vi "set_reference_object.vi"(1 "camera cluster":T2, 2 "bit depth":i32) -> (0 "last acquired buffer out":i32)   [LabVIEW 2010]
uses:
  <vilib>/userDefined/High Color/IMAQdx.ctl
  MWT_1.3.0_r1035/MultiWorm Tracker v1.3.0/data/MWT.dll
panel:
  in  "Store Reference Object from image":bool
  out "initial frame number":i32
  out "Reference Object Image":T3(plugin-control)
  in  "Reset":bool
  in  "Set":bool
  in  "Cancel":bool
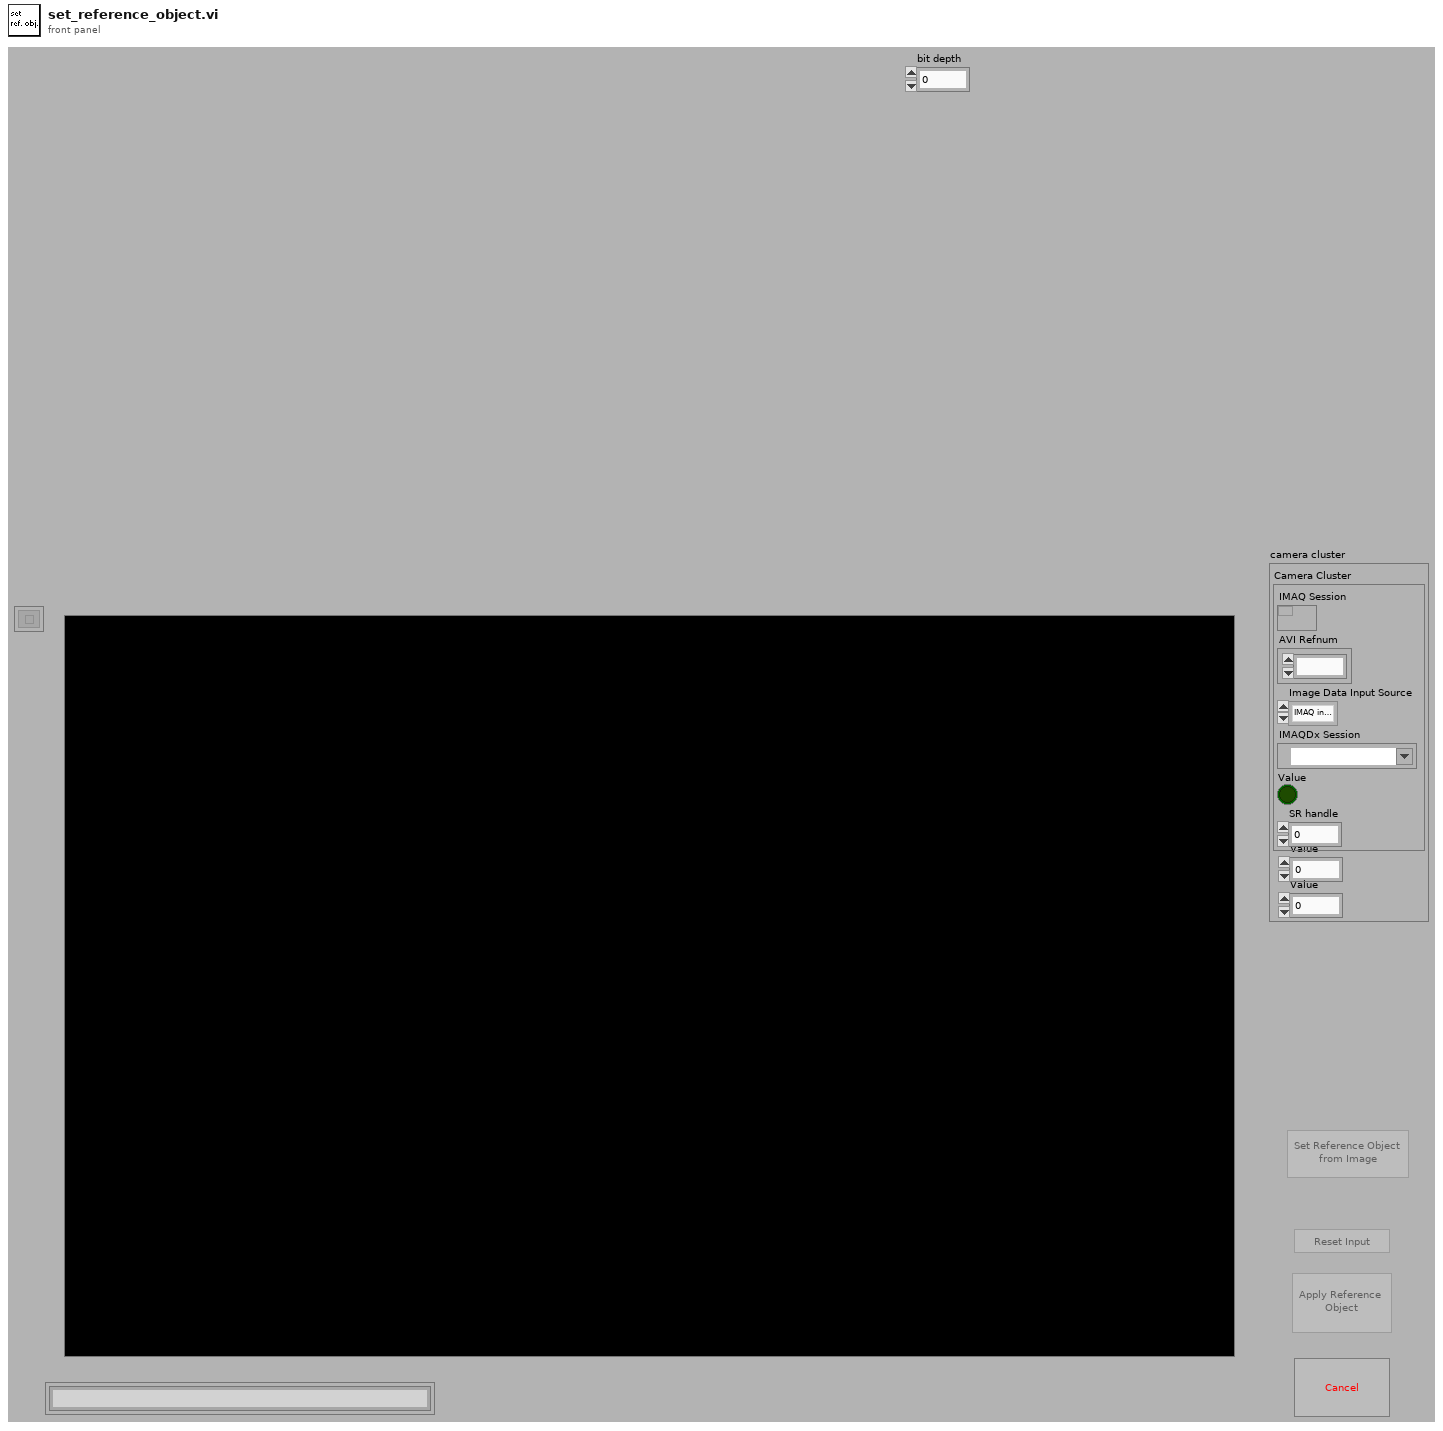
[diagram p1: front panel]
types:
  T1 = typedef "IMAQdx.ctl" = refnum<k21>
  T2 = cluster{"Camera Cluster":cluster{"IMAQ Session":refnum<k11>, "AVI Refnum":refnum<k1>, "Image Data Input Source":enum32{"IMAQ interface", "IMAQdx interface", "AVI file", "MMF File"}, "IMAQDx Session":T1, "Value":bool, "SR handle":u32}, "Value":i32, "Value":i32}
  T3 = typedef "IMAQ Image.ctl" = refnum<image>
  T4 = cluster{"Global Rectangle":i32[], "Contours":cluster{"Contour Type":u32, "ROI Type":u32, "Points":i32[]}[]}
  T5 = enum8{"Enabled", "Disabled", "Disabled and Grayed Out"}
  T6 = cluster{"IMAQ Session":refnum<k11>, "AVI Refnum":refnum<k1>, "Image Data Input Source":enum32{"IMAQ interface", "IMAQdx interface", "AVI file", "MMF File"}, "IMAQDx Session":T1, "Value":bool, "SR handle":u32}
  T7 = cluster{"Camera Cluster":cluster{"IMAQ Session":refnum<k11>, "AVI Refnum":refnum<k1>, "Image Data Input Source":enum32{"IMAQ interface", "IMAQdx interface", "AVI file", "MMF File"}, "IMAQDx Session":T1, "Value":bool, "SR handle":u32}, "Value":i32}
  T8 = cluster{"Camera Cluster":cluster{"IMAQ Session":refnum<k11>, "AVI Refnum":refnum<k1>, "Image Data Input Source":enum32{"IMAQ interface", "IMAQdx interface", "AVI file", "MMF File"}, "IMAQDx Session":T1, "Value":bool, "SR handle":u32}, "Acquired Buffer Number":i32}
  T9 = cluster{"Value":i32, i32, i32, "Image Pixels (I16)":i16[][]}
  T10 = cluster{"Value":i32, "Image Pixels (I16)":i16[][], "Image Pixels (I16)":i16[][], "Image Area Height":u32, "Image Area Width":u32}
  T11 = cluster{"return type":i32, "return type":i32, "destination":i16[][]}
  T12 = enum32{"IMAQ interface", "IMAQdx interface", "AVI file", "MMF File"}
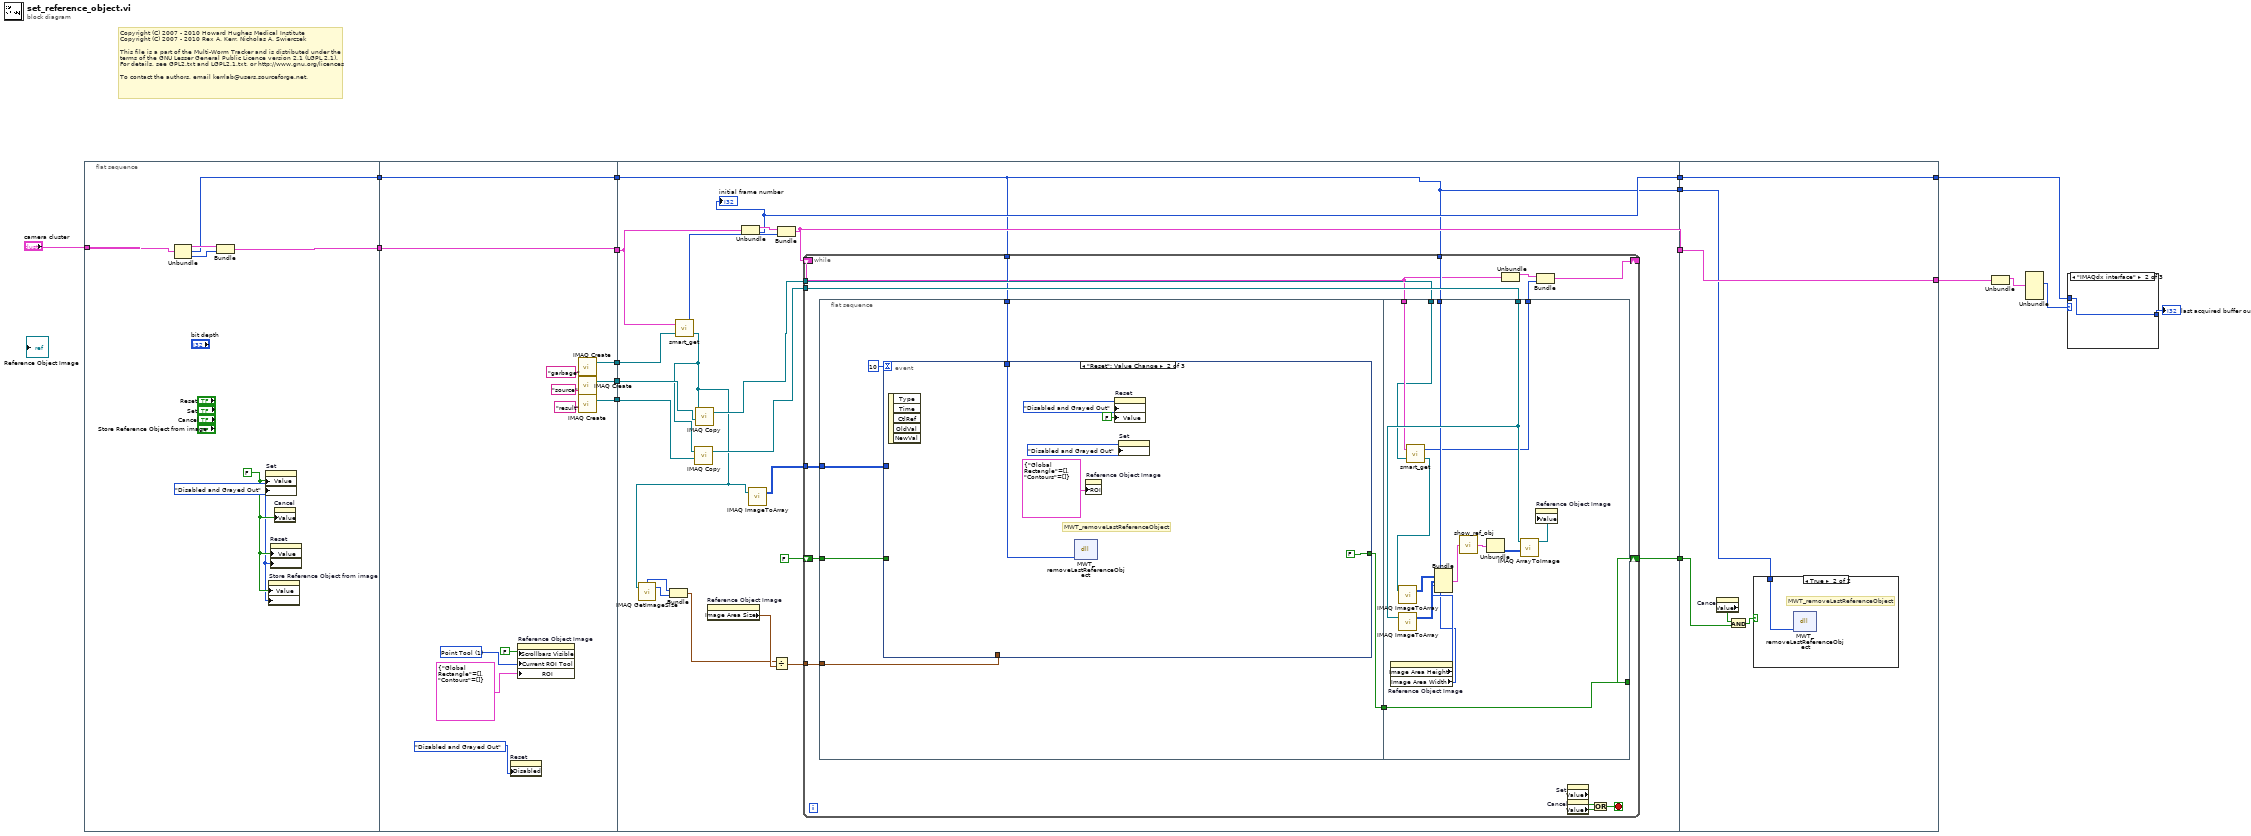
[diagram p0: block diagram]
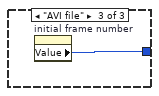
[diagram p3: hidden frame]
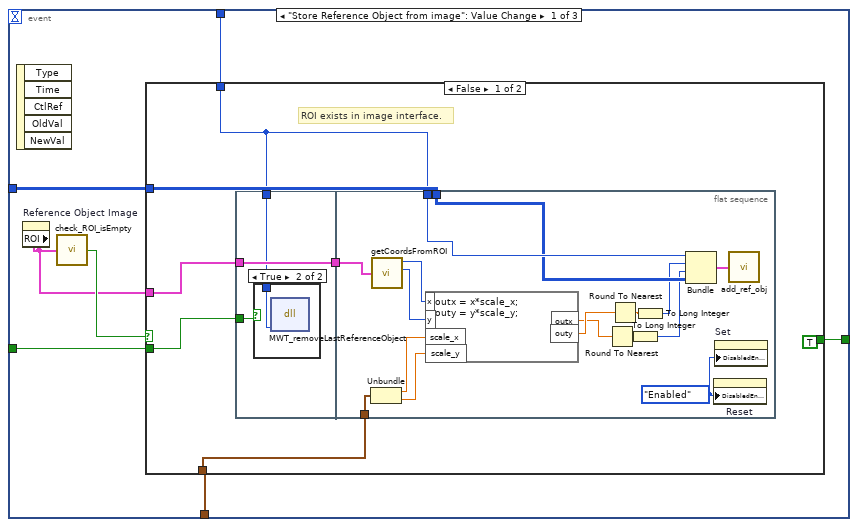
[diagram p4: hidden frame]
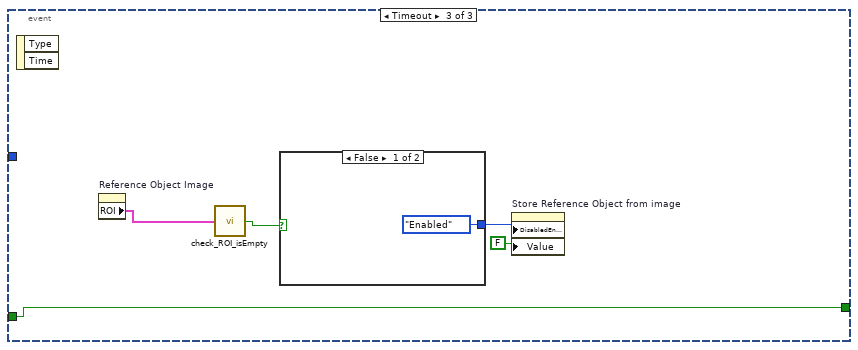
[diagram p7: hidden frame]
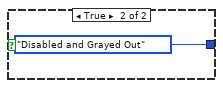
[diagram p8: hidden frame]
diagram:
  # "Copyright (C) 2007 - 2010 Howard Hughes Medical Institute\nCopyright (C) 2007 - 2010 Rex A. Kerr, Nicholas A. Swierczek\n \nThis file is a part of the Multi-Worm Tracker and is distributed under the\nterms of the GNU Lesser General Public Licence version 2.1 (LGPL 2.1).\nFor details, see GPL2.txt and LGPL2.1.txt, or http://www.gnu.org/licences\n \nTo contact the authors, email kerrlab@users.sourceforge.net."
  n1 = flat-sequence {
    tunnel: "camera cluster" -> [w24]
    tunnel: [w21] -> w17
    tunnel: [w20] -> w16
    tunnel: w17 -> [w31]
    tunnel: [w31] -> w14
    tunnel: [w35] -> w13
    tunnel: w16 -> [w35]
    tunnel: [w27] -> w6
    tunnel: [w26] -> w5
    tunnel: [w25] -> w4
    tunnel: w14 -> [w54]
    tunnel: w13 -> [w37]
    tunnel: [w53] -> w12
    tunnel: [w41] -> w11
    tunnel: w6 -> [w52]
    tunnel: w5 -> [w51]
    tunnel: w4 -> [w49]
    tunnel: [w38] -> w3
    tunnel: [w37] -> w2
    tunnel: w12 -> [w146]
    tunnel: w11 -> [w147]
    tunnel: [w147] -> w10
    tunnel: [w146] -> w7
    tunnel: w3 -> [w144]
    tunnel: w2 -> [w142]
    frame #0 {
      w18 = T5."Disabled and Grayed Out" ("Disabled")
      w19 = FALSE ("Set")
      n2 = Unbundle(w24) -> ("Camera Cluster"=w22:T6, "Value"=w20:i32, "Value"=w23:i32)
      n3 = Bundle("Camera Cluster"=w22, "Value"=w23) -> (w21:T7)  [unwired: 1 in]
      n4 = property on="Set" class="Bool (strict)"("Value"=w19, "DisabledEnum"=w18) -> ()  [unwired: 2 in, 2 out]
      n5 = property on="Store Reference Object from image" class="Bool (strict)"("Value"=w19, "DisabledEnum"=w18) -> ()  [unwired: 2 in, 2 out]
      n6 = property on="Reset" class="Bool (strict)"("Value"=w19, "DisabledEnum"=w18) -> ()  [unwired: 2 in, 2 out]
      n7 = property on="Cancel" class="Bool (strict)"("Value"=w19) -> ()  [unwired: 2 in, 2 out]
    }
    frame #1 {
      w34 = u32 1 items=["Zoom Tool"=8, "Selection Tool"=0, "Pan Tool"=9, "Point Tool"=1, "Line Tool"=2, "Rectangle Tool"=3, "Rotated Rectangle Tool"=12, "Polyline Tool"=10, "Polygon Tool"=5, "Freehand Tool"=11, "Closed Freehand Tool"=6, "Ellipse Tool"=4, "Annulus Tool"=7] ("Current ROI Tool")
      n8 = property on="Reset" class="Bool (strict)"("Disabled"=T5."Disabled and Grayed Out") -> ()  [unwired: 2 in, 2 out]
      n9 = property on="Reference Object Image" class="ImageControl"("Scrollbars Visible"=FALSE, "Current ROI Tool"=w34, "ROI"=T4 {"Global Rectangle"=[], "Contours"=[]}) -> ()  [unwired: 2 in, 2 out]
      n10 = call "IMAQ Create"("Image Name"="garbage") -> ("New Image"=w27:T3)  [unwired: 4 in, 1 out]
      n11 = call "IMAQ Create"("Image Name"="source") -> ("New Image"=w25:T3)  [unwired: 4 in, 1 out]
      n12 = call "IMAQ Create"("Image Name"="result") -> ("New Image"=w26:T3)  [unwired: 4 in, 1 out]
    }
    frame #2 {
      n13 = call "smart_get.vi"("Input Image"=w52, "Cluster"=w54) -> ("Image Out"=w43:T3, "Acquired Buffer Number"=w56:i32)
      n14 = call "IMAQ GetImageSize"("Image"=w43) -> ("Y Resolution"=w44:i32, "X Resolution"=w45:i32)  [unwired: 3 in, 1 out]
      n15 = Bundle("X Resolution"=w45, "Y Resolution"=w44) -> (w39:cluster{"X Resolution":i32, "Y Resolution":i32})  [unwired: 1 in]
      n16 = call "IMAQ Copy"("Image Dst"=w51, "Image Src"=w43) -> ("Image Dst Out"=w50:T3)  [unwired: 4 in, 1 out]
      n17 = call "IMAQ Copy"("Image Dst"=w49, "Image Src"=w43) -> ("Image Dst Out"=w48:T3)  [unwired: 4 in, 1 out]
      n18 = property on="Reference Object Image" class="ImageControl"() -> ("Image Area Size"=w40:cluster{"Width":u32, "Height":u32})  [unwired: 2 in, 2 out]
      n19 = Unbundle(w54) -> ("Camera Cluster"=w55:T6, "Value"=w53:i32)
      "initial frame number" <- w53
      n20 = call "IMAQ ImageToArray"("Image"=w43) -> ("Image Pixels (I16)"=w46:i16[][])  [unwired: 3 in, 4 out]
      n21 = Divide(x=w39, y=w40) -> (x/y=w42:cluster{dbl, dbl})
      n22 = Bundle("Camera Cluster"=w55, "Acquired Buffer Number"=w56) -> (w41:T8)  [unwired: 1 in]
      n23 = while {
        tunnel: w50 -> [w69]
        tunnel: w48 -> [w68]
        tunnel: w37 -> [w67]
        shift-right: [w64] -> w38
        shift-left: FALSE -> [w66]
        tunnel: w37 -> [w63]
        tunnel: w46 -> [w62]
        tunnel: w42 -> [w61]
        shift-right: [w57] -> _
        shift-left: w41 -> [w59]
        stop <- w70 stop-if-true
        n24 = flat-sequence {
          tunnel: w66 -> [w77]
          tunnel: [w76] -> w65
          tunnel: w63 -> [w75]
          tunnel: w62 -> [w74]
          tunnel: w61 -> [w73]
          tunnel: w69 -> [w138]
          tunnel: w68 -> [w128]
          tunnel: w67 -> [w137]
          tunnel: w65 -> [w131]
          tunnel: [w131] -> w64
          tunnel: w59 -> [w130]
          tunnel: [w129] -> w58
          frame #0 {
            n25 = event shown="[1] \"Reset\": Value Change" {
              selector: _ -> [_ _ _]
              dyn-events: _ -> [_ _ _]
              timeout: 10 -> [_ _ _]
              tunnel: w77 -> [w84 _ w124]
              tunnel: [w83 FALSE w124] -> w76
              tunnel: w75 -> [w81 w118 _]
              tunnel: w74 -> [w80 _ _]
              tunnel: w73 -> [w79 _ _]
              event "Store Reference Object from image": Value Change {
                n26 = event-data() -> ()  [unwired: 1 in, 5 out]
                n27 = property on="Reference Object Image" class="ImageControl"() -> ("ROI"=w82:T4)  [unwired: 2 in, 2 out]
                n28 = call "check_ROI_isEmpty.vi"("ROI"=w82) -> ("empty?"=w85:bool)
                n29 = case shown="False" w85 {
                  tunnel: w84 -> [w86 w113]
                  tunnel: [TRUE w113] -> w83
                  tunnel: w82 -> [w91 _]
                  tunnel: w81 -> [w87 _]
                  tunnel: w80 -> [w90 _]
                  tunnel: w79 -> [w89 _]
                  frame False {
                    # "ROI exists in image interface."
                    n30 = flat-sequence {
                      tunnel: w91 -> [w95]
                      tunnel: [w95] -> w88
                      tunnel: w87 -> [w94]
                      tunnel: w86 -> [w93]
                      tunnel: w87 -> [w111]
                      tunnel: w90 -> [w110]
                      tunnel: w89 -> [w109]
                      tunnel: w88 -> [w112]
                      frame #0 {
                        n31 = case shown="True" w93 {
                          tunnel: w94 -> [_ w96]
                          frame False {
                          }
                          frame True {
                            n32 = dll-call lib="C:/Users/Marc/multi worm tracker/MWT_1.3.0_r1035/MultiWorm Tracker v1.3.0/data/MWT.dll" fn="MWT_removeLastReferenceObject"("handle"=w96) -> ()  [unwired: 5 in, 2 out]
                          }
                        }
                      }
                      frame #1 {
                        w97 = T5."Enabled" ("Disabled")
                        n33 = Unbundle(w109) -> (w101:dbl, w100:dbl)
                        n34 = call "getCoordsFromROI.vi"("ROI"=w112) -> ("y1"=w102:i32, "x1"=w103:i32)  [unwired: 2 out]
                        n35 = formula code="outx = x*scale_x;\nouty = y*scale_y;"("x"=w103, "y"=w102, "scale_x"=w101, "scale_y"=w100) -> ("outx"=w98:dbl, "outy"=w99:dbl)
                        n36 = Round To Nearest(number=w98) -> (nearest integer value=w104:dbl)
                        n37 = Round To Nearest(number=w99) -> (nearest integer value=w105:dbl)
                        n38 = To Long Integer(number=w104) -> (32bit integer=w107:i32)
                        n39 = To Long Integer(number=w105) -> (32bit integer=w106:i32)
                        n40 = Bundle("Value"=w111, w106, w107, "Image Pixels (I16)"=w110) -> (w108:T9)  [unwired: 1 in]
                        n41 = property on="Reset" class="Bool (strict)"("DisabledEnum"=w97) -> ()  [unwired: 2 in, 2 out]
                        n42 = property on="Set" class="Bool (strict)"("DisabledEnum"=w97) -> ()  [unwired: 2 in, 2 out]
                        n43 = call "add_ref_obj.vi"("input cluster"=w108) -> ()  [unwired: 1 out]
                      }
                    }
                  }
                  frame True {
                    # "No ROI set in image interface.\nDo nothing."
                  }
                }
              }
              event "Reset": Value Change {
                # "MWT_removeLastReferenceObject"
                n44 = event-data() -> ()  [unwired: 1 in, 5 out]
                n45 = dll-call lib="C:/Users/Marc/multi worm tracker/MWT_1.3.0_r1035/MultiWorm Tracker v1.3.0/data/MWT.dll" fn="MWT_removeLastReferenceObject"("handle"=w118) -> ()  [unwired: 5 in, 2 out]
                n46 = property on="Reference Object Image" class="ImageControl"("ROI"=T4 {"Global Rectangle"=[], "Contours"=[]}) -> ()  [unwired: 2 in, 2 out]
                n47 = property on="Reset" class="Bool (strict)"("DisabledEnum"=T5."Disabled and Grayed Out" ("Disabled"), "Value"=FALSE ("Reset")) -> ()  [unwired: 2 in, 2 out]
                n48 = property on="Set" class="Bool (strict)"("DisabledEnum"=T5."Disabled and Grayed Out" ("Disabled")) -> ()  [unwired: 2 in, 2 out]
              }
              event Timeout {
                n49 = event-data() -> ()  [unwired: 1 in, 2 out]
                n50 = property on="Reference Object Image" class="ImageControl"() -> ("ROI"=w123:T4)  [unwired: 2 in, 2 out]
                n51 = call "check_ROI_isEmpty.vi"("ROI"=w123) -> ("empty?"=w122:bool)
                n52 = case shown="False" w122 {
                  tunnel: [T5."Enabled" ("Disabled") T5."Disabled and Grayed Out" ("Disabled")] -> w121
                  frame False {
                  }
                  frame True {
                  }
                }
                n53 = property on="Store Reference Object from image" class="Bool (strict)"("DisabledEnum"=w121, "Value"=FALSE ("Store Reference Object from image")) -> ()  [unwired: 2 in, 2 out]
              }
            }
          }
          frame #1 {
            n54 = property on="Reference Object Image" class="ImageControl"() -> ("Image Area Height"=w134:u32, "Image Area Width"=w133:u32)  [unwired: 2 in, 2 out]
            n55 = call "IMAQ ImageToArray"("Image"=w138) -> ("Image Pixels (I16)"=w135:i16[][])  [unwired: 3 in, 4 out]
            n56 = call "smart_get.vi"("Input Image"=w128, "Cluster"=w130) -> ("Image Out"=w127:T3, "Acquired Buffer Number"=w129:i32)
            n57 = call "IMAQ ImageToArray"("Image"=w127) -> ("Image Pixels (I16)"=w136:i16[][])  [unwired: 3 in, 4 out]
            n58 = Bundle("Value"=w137, "Image Pixels (I16)"=w136, "Image Pixels (I16)"=w135, "Image Area Height"=w134, "Image Area Width"=w133) -> (w132:T10)  [unwired: 1 in]
            n59 = call "show_ref_obj.vi"("input cluster"=w132) -> ("output cluster"=w141:T11)
            n60 = Unbundle(w141) -> ("destination"=w140:i16[][])  [unwired: 2 out]
            n61 = call "IMAQ ArrayToImage"("Image Pixels (I16)"=w140, "Image"=w138) -> ("Image Out"=w139:T3)  [unwired: 8 in, 1 out]
            n62 = property on="Reference Object Image" class="ImageControl"("Value"=w139) -> ()  [unwired: 2 in, 2 out]
          }
        }
        n63 = Unbundle(w59) -> ("Camera Cluster"=w60:T6)  [unwired: 1 out]
        n64 = Bundle("Camera Cluster"=w60, "Acquired Buffer Number"=w58) -> (w57:T8)  [unwired: 1 in]
        n65 = property on="Set" class="Bool (strict)"() -> ("Value"=w72:bool)  [unwired: 2 in, 2 out]
        n66 = property on="Cancel" class="Bool (strict)"() -> ("Value"=w71:bool)  [unwired: 2 in, 2 out]
        n67 = Or(x=w72, y=w71) -> (x .or. y?=w70:bool)
      }
    }
    frame #3 {
      n68 = property on="Cancel" class="Bool (strict)"() -> ("Value"=w145:bool)  [unwired: 2 in, 2 out]
      n69 = And(x=w145, y=w144) -> (x .and. y?=w143:bool)
      n70 = case shown="True" w143 {
        tunnel: w142 -> [_ w148]
        frame False {
        }
        frame True {
          # "MWT_removeLastReferenceObject"
          n71 = dll-call lib="C:/Users/Marc/multi worm tracker/MWT_1.3.0_r1035/MultiWorm Tracker v1.3.0/data/MWT.dll" fn="MWT_removeLastReferenceObject"("handle"=w148) -> ()  [unwired: 5 in, 2 out]
        }
      }
    }
  }
  n72 = Unbundle(w10) -> ("Camera Cluster"=w9:T6)  [unwired: 1 out]
  n73 = Unbundle(w9) -> ("Image Data Input Source"=w8:T12)  [unwired: 5 out]
  n74 = case shown="\"IMAQdx interface\"" w8 {
    tunnel: [w149 w150 w151] -> w15
    tunnel: w7 -> [w149 w150 _]
    frame "IMAQ interface", Default {
    }
    frame "IMAQdx interface" {
    }
    frame "AVI file" {
      n75 = property on="initial frame number" class="DigNum (strict)"() -> ("Value"=w151:i32)  [unwired: 2 in, 2 out]
    }
  }
  "last acquired buffer out" <- w15
